vi "ChangeInheritance.vi"(0 "ClassWriterGOOP300 in":refnum<class "ClassWriterGOOP300.lvclass">, 1 "LvClass":refnum<vi>, 2 "NewBaseClass(Empty=ConvertClassToBaseClass)":path=path "C:/Documents and Settings/Micke/Skrivbord/My Computer/B_class/B.lvclass", 5 "error in (no error)":errorcluster) -> (14 "ClassWriterGOOP300 out":refnum<class "ClassWriterGOOP300.lvclass">, 19 "error out":errorcluster)   [LabVIEW 2012, in "ClassWriterGOOP300.lvclass"]
uses:
  <resource>/Framework/Providers/Open_GDS/ClassProviders/Provider_EndevoGOOP300/ClassWriterGOOP300_class/ClassWriterGOOP300.lvclass
  <resource>/Framework/Providers/Open_GDS/ClassProviders/Provider_EndevoGOOP300/Templates/EndevoTemplateNames.ctl
  <resource>/Framework/Providers/Open_GDS/ClassProviders/Provider_LvNativeClass/ClassWriterNative_class/ClassWriterNative.lvclass
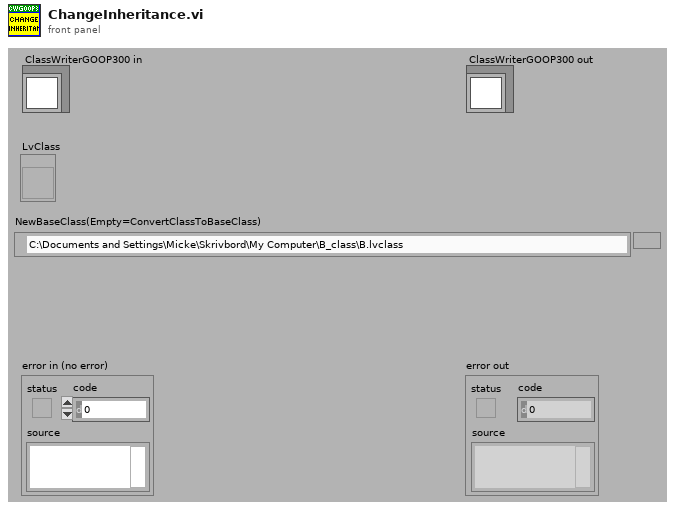
[diagram p1: front panel]
types:
  T1 = typedef "EndevoTemplateNames.ctl" = enum16{"BaseTemplate", "SubTemplate", "BaseTemplate_4x4x4", "SubTemplate_4x4x4", "SingletonTemplate"}
  T2 = typedef "GDSLvCLass_ClassSettingsType.ctl" = cluster{"ClassProviderName":string, "ClassTemplateUsed":string, "ClassTemplateVersion":string, "ClassDescription":string, "PlugIns":T3[], "ConnectorPanePattern":string}
  T3 = typedef "GDSLvClass_PlugIn.ctl" = cluster{"Type":T4, "ID":string, "Version":string, "Path":path, "Name":string, "Data":variant}
  T4 = typedef "GDSLvClass_PlugInTypes.ctl" = enum16{"DesignPattern", "MethodTypes"}
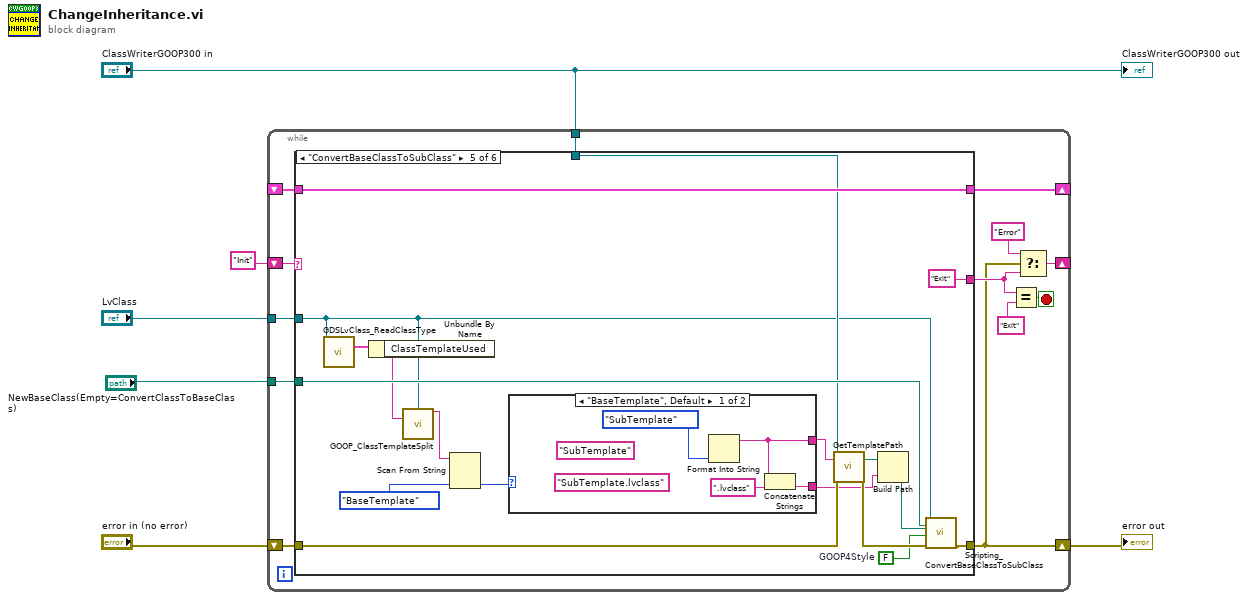
[diagram p0: block diagram]
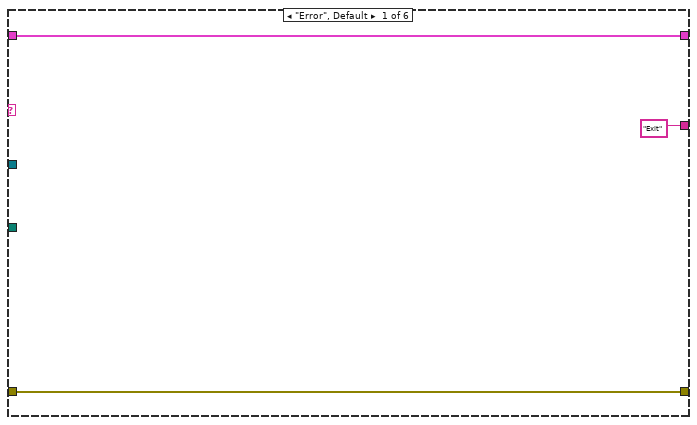
[diagram p2: hidden frame]
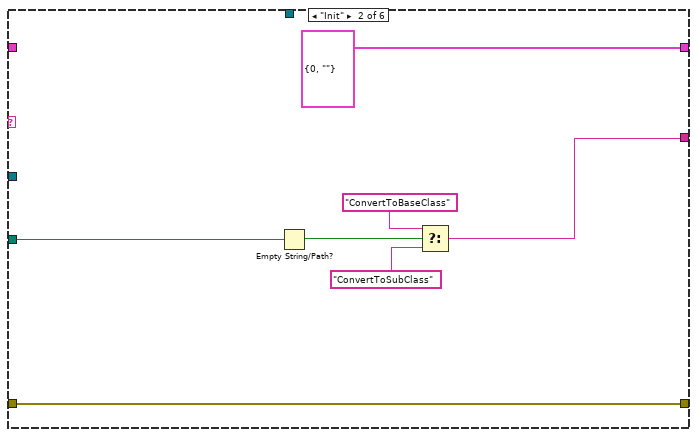
[diagram p3: hidden frame]
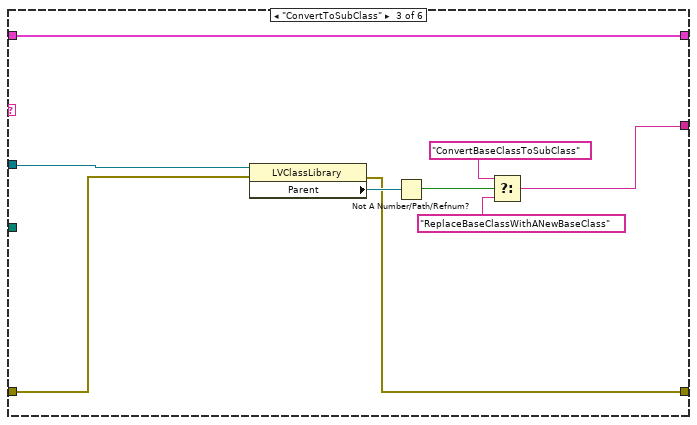
[diagram p4: hidden frame]
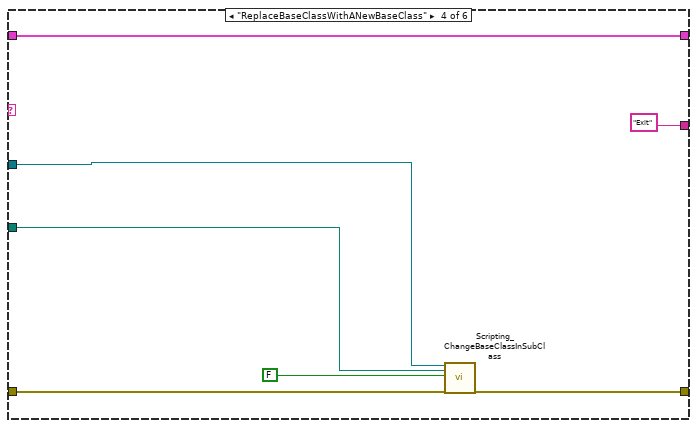
[diagram p5: hidden frame]
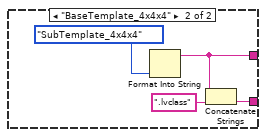
[diagram p6: hidden frame]
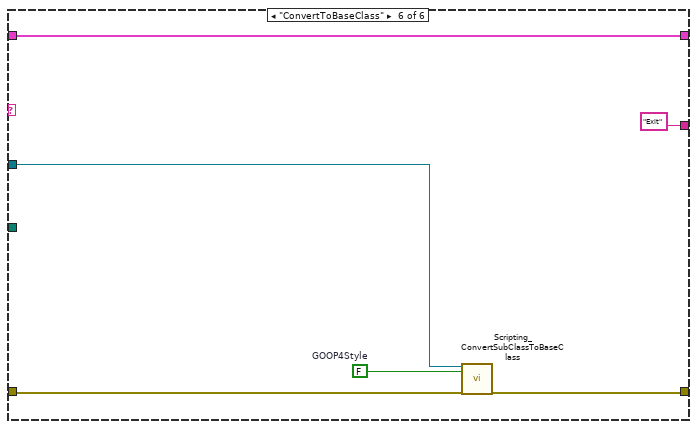
[diagram p7: hidden frame]
diagram:
  n1 = while {
    shift-right: [w13] -> w4
    shift-left: "error in (no error)" -> [w19]
    shift-right: [w17] -> _
    shift-left: "Init" -> [w18]
    shift-right: [w12] -> _
    shift-left: _ -> [w11]
    tunnel: "NewBaseClass(Empty=ConvertClassToBaseClass)" -> [w10]
    tunnel: "LvClass" -> [w9]
    tunnel: "ClassWriterGOOP300 in" -> [w7]
    stop <- w16 stop-if-true
    n2 = case shown="\"ConvertBaseClassToSubClass\"" w18 {
      tunnel: w19 -> [w22 w29 w37 w43 w61 w75]
      tunnel: [w22 w29 w32 w42 w63 w73] -> w13
      tunnel: ["Exit" w24 w33 "Exit" "Exit" "Exit"] -> w14
      tunnel: [w20 cluster{"Counter":i32, "Text":string} {"Counter"=0, "Text"=""} w30 w45 w56 w77] -> w12
      tunnel: w11 -> [w20 _ w30 w45 w56 w77]
      tunnel: w10 -> [_ w27 _ w40 w62 _]
      tunnel: w9 -> [_ _ w38 w41 w46 w74]
      tunnel: w7 -> [_ _ _ _ w55 _]
      frame "Error", Default {
      }
      frame "Init" {
        n3 = Empty String/Path?(string/path=w27) -> (empty?=w26:bool)
        n4 = Select(t="ConvertToBaseClass", s=w26, f="ConvertToSubClass") -> (s? t:f=w24:string)
      }
      frame "ConvertToSubClass" {
        n5 = property class="LVClassLibrary"(reference=w38, error in=w37) -> (error out=w32:errorcluster, "Parent"=w36:refnum<vi>)  [unwired: 1 out]
        n6 = Not A Number/Path/Refnum?(number/path/refnum=w36) -> (NaN/Path/Refnum?=w35:bool)
        n7 = Select(t="ConvertBaseClassToSubClass", s=w35, f="ReplaceBaseClassWithANewBaseClass") -> (s? t:f=w33:string)
      }
      frame "ReplaceBaseClassWithANewBaseClass" {
        n8 = call <resource>:"Scripting_ChangeBaseClassInSubClass.vi"("SubClass"=w41, "NewBaseClass"=w40, "GOOP4Style"=FALSE, "error in (no error)"=w43) -> ("error out"=w42:errorcluster)  [unwired: 15 in]
      }
      frame "ConvertBaseClassToSubClass" {
        w49 = FALSE  # GOOP4Style
        n9 = call <resource>:"GDSLvClass_ReadClassType.vi"("Class Refnum In"=w46) -> ("ClassSettings"=w52:T2)  [unwired: 16 in, 2 out]
        n10 = Unbundle By Name(w52) -> ("ClassTemplateUsed"=w47:string)
        n11 = call <resource>:"GOOP_ClassTemplateSplit.vi"("ClassItemRefIn"=w46, "FullClassTemplate"=w47) -> ("StandardTemplate"=w48:string)  [unwired: 12 in, 1 out]
        n12 = Scan From String(input string=w48, default 1=EndevoTemplateNames."BaseTemplate" ("TemplateNames")) -> (output 1=w54:T1)  [unwired: 3 in, 3 out]
        n13 = case shown="\"BaseTemplate\", Default" w54 {
          tunnel: [w65 w69] -> w51
          tunnel: [w66 w70] -> w50
          frame "BaseTemplate", Default {
            (unwired) "SubTemplate.lvclass" ("name or relative path")
            (unwired) "SubTemplate" ("ClassTemplateSubDirectory")
            n14 = Format Into String(EndevoTemplateNames."SubTemplate" ("TemplateNames")) -> (resulting string=w65:string)  [unwired: 3 in, 1 out]
            n15 = Concatenate Strings(w65, ".lvclass" ("name or relative path")) -> (w66:string)
          }
          frame "BaseTemplate_4x4x4" {
            n16 = Format Into String(EndevoTemplateNames."SubTemplate_4x4x4" ("TemplateNames")) -> (resulting string=w69:string)  [unwired: 3 in, 1 out]
            n17 = Concatenate Strings(w69, ".lvclass" ("name or relative path")) -> (w70:string)
          }
        }
        n18 = call-dynamic "GetTemplatePath.vi"("reference in"=w55, "ClassTemplateSubDirectory"=w51, "error in (no error)"=w61) -> ("FolderPathOut"=w59:path, "error out"=w60:errorcluster)  [unwired: 12 in, 3 out]
        n19 = Build Path(base path=w59, name or relative path=w50) -> (appended path=w58:path)
        n20 = call <resource>:"Scripting_ConvertBaseClassToSubClass.vi"("BaseClass"=w46, "NewBaseClass"=w62, "SubClassTemplate"=w58, "GOOP4Style"=w49, "error in (no error)"=w60) -> ("error out"=w63:errorcluster)  [unwired: 14 in]
      }
      frame "ConvertToBaseClass" {
        w72 = FALSE  # GOOP4Style
        n21 = call <resource>:"Scripting_ConvertSubClassToBaseClass.vi"("SubClass"=w74, "GOOP4Style"=w72, "error in (no error)"=w75) -> ("error out"=w73:errorcluster)  [unwired: 16 in]
      }
    }
    n22 = Equal?(x=w14, y="Exit") -> (x = y?=w16:bool)
    n23 = Select(t="Error", s=w13, f=w14) -> (s? t:f=w17:string)
  }
  "error out" <- w4
  "ClassWriterGOOP300 out" <- "ClassWriterGOOP300 in"
